vi "Actual Flow.vi"(8 "Error In":errorcluster, 10 "Channel (0)":i32, 11 "VISA resource name":refnum<visa-resource-name>) -> (0 "Error Out":errorcluster, 1 "Actual Flow":dbl, 3 "dup VISA resource name":refnum<visa-resource-name>)   [LabVIEW 2011, in "MGC647C.lvlib"]
doc: "Read actual flow of a channel."
uses:
  <instrlib>/MGC647C/MGC647C.lvlib
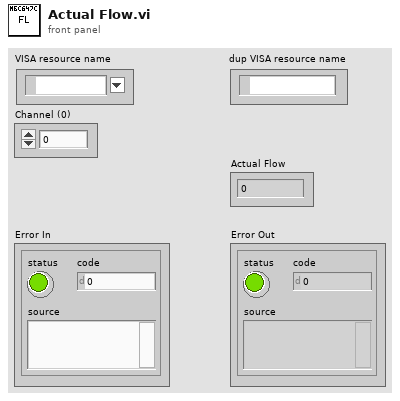
[diagram p1: front panel]
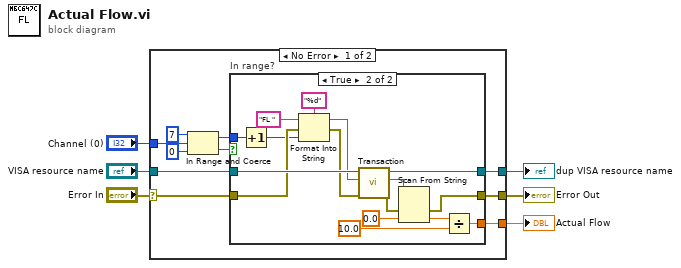
[diagram p0: block diagram]
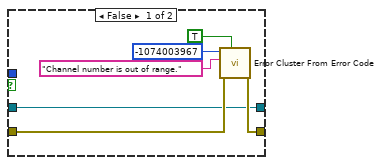
[diagram p2: hidden frame]
diagram:
  n1 = case shown="No Error" "Error In" {
    selector: "Error In" -> [w13 w40]
    tunnel: "VISA resource name" -> [w16 w39]
    tunnel: [w15 w39] -> w5
    tunnel: [w14 w40] -> w4
    tunnel: [w12 _] -> w2
    tunnel: "Channel (0)" -> [w9 _]
    frame No Error {
      n2 = In Range and Coerce(upper limit=7, x=w9, lower limit=0) -> (coerced(x)=w8:i32, In Range?=w7:bool)
      n3 = case "In range?" shown="True" w7 {
        tunnel: w16 -> [w20 w38]
        tunnel: [w20 w37] -> w15
        tunnel: [w21 w32] -> w14
        tunnel: w13 -> [w22 w36]
        tunnel: [_ w28] -> w12
        tunnel: w8 -> [_ w30]
        frame False {
          n4 = call <vilib>:"Error Cluster From Error Code.vi"("show call chain? (False)"=TRUE, "error in (no error)"=w22, "error message (\"\")"="Channel number is out of range." ("error message (\"\")"), "error code (0)"=-1074003967) -> ("error out"=w21:errorcluster)  [unwired: 5 in]
        }
        frame True {
          n5 = Increment(x=w30) -> (x+1=w29:i32)
          n6 = Format Into String(format string="%d", initial string="FL " ("string (\"\")"), error in=w36, w29) -> (resulting string=w25:string, error out=w35:errorcluster)
          n7 = call <instrlib>:"Transaction.vi"("Error In"=w35, "Command"=w25, "VISA resource name"=w38) -> ("Error Out"=w33:errorcluster, "Response"=w34:string, "dup VISA resource name"=w37:refnum<visa-resource-name>)  [unwired: 6 in]
          n8 = Scan From String(input string=w34, error in=w33, default 1=0.0 ("default value 1")) -> (error out=w32:errorcluster, output 1=w31:dbl)  [unwired: 2 in, 2 out]
          n9 = Divide(x=w31, y=10.0) -> (x/y=w28:dbl)
        }
      }
    }
    frame Error {
    }
  }
  "dup VISA resource name" <- w5
  "Error Out" <- w4
  "Actual Flow" <- w2
